vi "view network stream messages.vi"(9 "RT status":T2, 11 "Array":T1[](array[typedef])) -> (1 "RT status":T2, 3 "Array out":T1[](array[typedef]))   [LabVIEW 2018]
uses:
  RT/Type Defs/generic incident.ctl
  RT/Type Defs/RT Status.ctl
  RT/Type Defs/warning incident cluster.ctl
  RT/Type Defs/error incident cluster.ctl
panel:
  out "Array 4":errorcluster[](array[cluster])
  out "call chain":string[][](array[string])
  out "error description":string[](array[string])
  out "Array 3":string[](array[string])
  out "Array 2":timestamp[](array[timestamp])
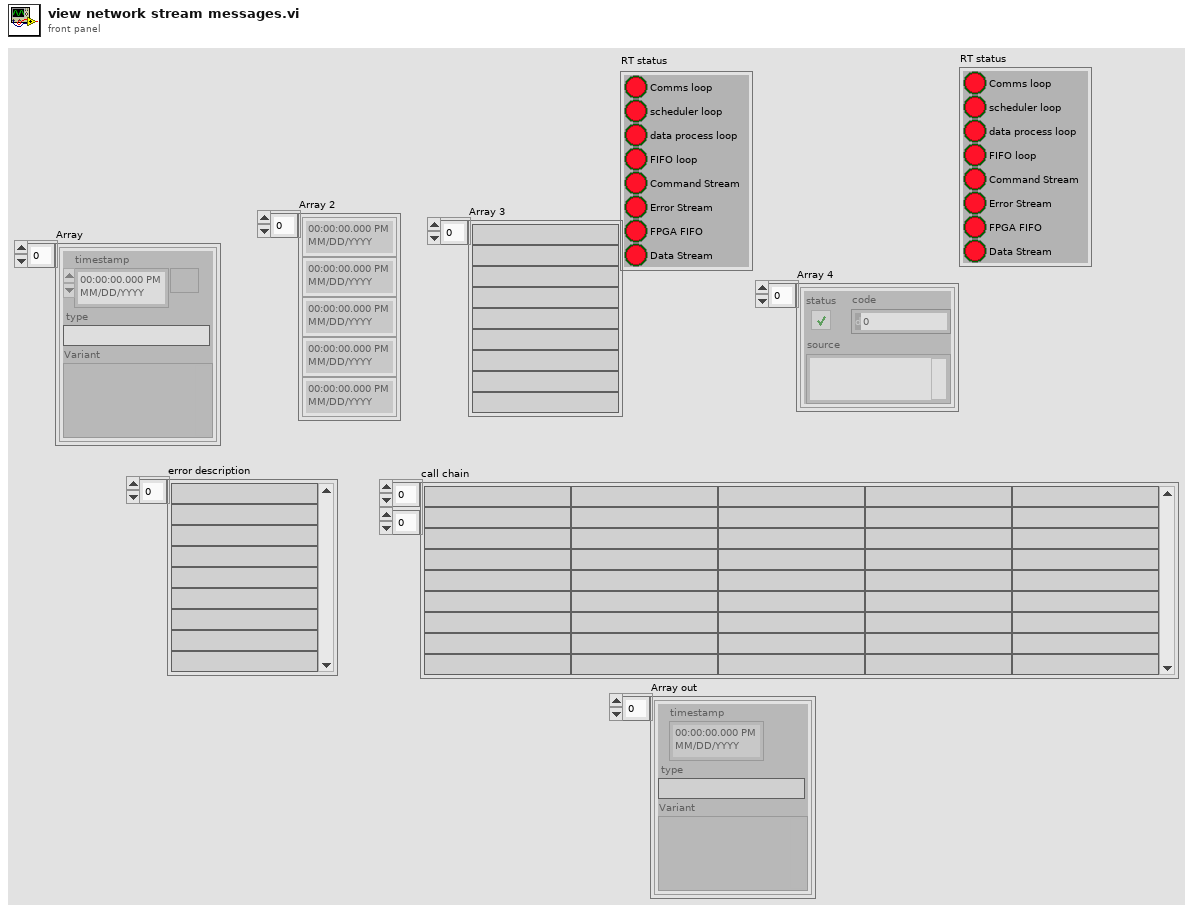
[diagram p1: front panel]
types:
  T1 = typedef "generic incident.ctl" = cluster{"timestamp":timestamp, "type":string, "Variant":variant}
  T2 = typedef "RT Status.ctl" = cluster{"Comms loop":bool, "scheduler loop":bool, "data process loop":bool, "FIFO loop":bool, "Command Stream":bool, "Error Stream":bool, "FPGA FIFO":bool, "Data Stream":bool}
  T3 = typedef "warning incident cluster.ctl" = cluster{"warning description":string, "call chain":string[]}
  T4 = typedef "error incident cluster.ctl" = cluster{"description":string, "call chain":string[], "error":errorcluster}
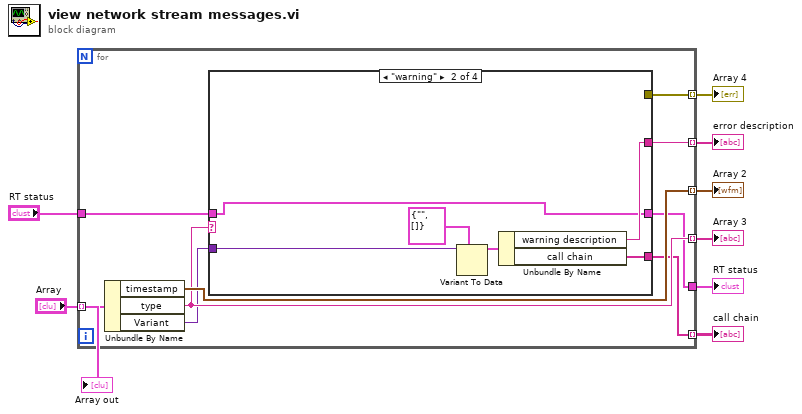
[diagram p0: block diagram]
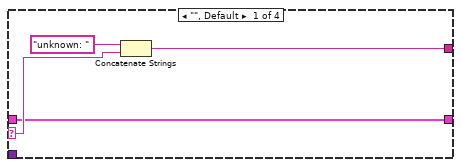
[diagram p2: hidden frame]
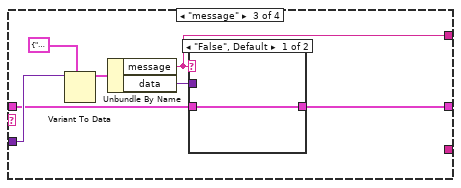
[diagram p3: hidden frame]
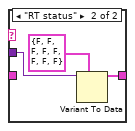
[diagram p4: hidden frame]
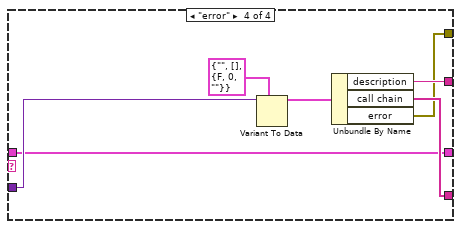
[diagram p5: hidden frame]
diagram:
  n1 = for {
    tunnel: "Array" -> [w17] mode=indexing
    tunnel: [w16] -> w7 mode=indexing
    tunnel: [w15] -> w6 mode=indexing
    tunnel: [w13] -> w5 mode=indexing
    tunnel: [w12] -> w4 mode=indexing
    tunnel: [w11] -> w3 mode=indexing
    tunnel: [w10] -> w2
    tunnel: "RT status" -> [w9]
    n2 = Unbundle By Name(w17) -> ("timestamp"=w16:timestamp, "type"=w15:string, "Variant"=w14:variant)
    n3 = case shown="\"warning\"" w15 {
      selector: w15 -> [w21 _ _ _]
      tunnel: w14 -> [_ w27 w34 w45]
      tunnel: [w20 w24 w31 w42] -> w13
      tunnel: [_ w23 _ w41] -> w12
      tunnel: [_ _ _ w40] -> w11
      tunnel: [w18 w22 w29 w39] -> w10
      tunnel: w9 -> [w18 w22 w28 w39]
      frame "", Default {
        n4 = Concatenate Strings("unknown: " ("string"), w21) -> (w20:string)
      }
      frame "warning" {
        n5 = Variant To Data(type=T3 {"warning description"="", "call chain"=[]} ("cluster"), Variant=w27) -> (data=w25:T3)  [unwired: 1 in, 1 out]
        n6 = Unbundle By Name(w25) -> ("warning description"=w24:string, "call chain"=w23:string[])
      }
      frame "message" {
        n7 = Variant To Data(type=cluster{"message":string, "data":variant} {"message"="", "data"=variant}, Variant=w34) -> (data=w32:cluster{"message":string, "data":variant})  [unwired: 1 in, 1 out]
        n8 = Unbundle By Name(w32) -> ("message"=w31:string, "data"=w30:variant)
        n9 = case shown="\"False\", Default" w31 {
          tunnel: w30 -> [_ w38]
          tunnel: [w35 w36] -> w29
          tunnel: w28 -> [w35 _]
          frame "False", Default {
          }
          frame "RT status" {
            n10 = Variant To Data(type=T2 {"Comms loop"=FALSE, "scheduler loop"=FALSE, "data process loop"=FALSE, "FIFO loop"=FALSE, "Command Stream"=FALSE, "Error Stream"=FALSE, "FPGA FIFO"=FALSE, "Data Stream"=FALSE} ("RT Status"), Variant=w38) -> (data=w36:T2)  [unwired: 1 in, 1 out]
          }
        }
      }
      frame "error" {
        n11 = Variant To Data(type=T4 {"description"="", "call chain"=[], "error"={"status"=FALSE, "code"=0, "source"=""}} ("cluster"), Variant=w45) -> (data=w43:T4)  [unwired: 1 in, 1 out]
        n12 = Unbundle By Name(w43) -> ("description"=w42:string, "call chain"=w41:string[], "error"=w40:errorcluster)
      }
    }
  }
  "Array 2" <- w7
  "Array 3" <- w6
  "error description" <- w5
  "call chain" <- w4
  "Array 4" <- w3
  "RT status" <- w2
  "Array out" <- "Array"
